vi "FormatInput.vi"(6 "Count to skip":u32, 7 "reset":bool, 8 "valid in":bool, 10 "factor":u16, 11 "data in":T1[](array[typedef])=[{"I"=0.0, "Q"=0.0, "overflow"=FALSE}, {"I"=0.0, "Q"=0.0, "overflow"=FALSE}]) -> (0 "valid out":bool, 3 "Array out":T2)   [LabVIEW 2025]
uses:
  FPGA/subVIs/I32 array size 4.ctl
  <instrlib>/_niInstr/DSP/v1/Shared/Public/IQ Data.ctl
  <instrlib>/_niInstr/DSP/v1/Shared/niInstr DSP v1 Shared.lvlib
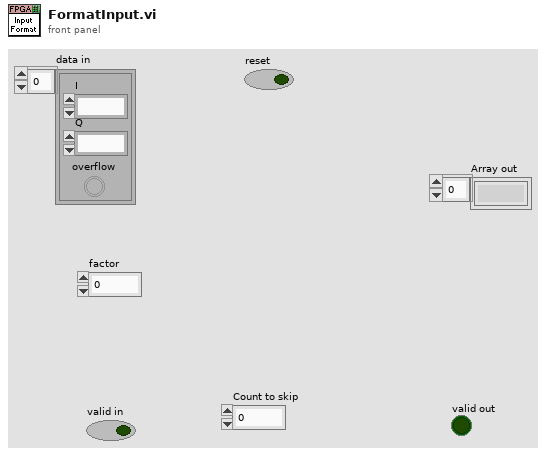
[diagram p1: front panel]
types:
  T1 = typedef "niInstr DSP v1 Shared.lvlib/IQ Data.ctl" = cluster{"I":fxp<+/-,18,1>, "Q":fxp<+/-,18,1>, "overflow":bool}
  T2 = typedef "I32 array size 4.ctl" = fxp<+/-,32,14>[]
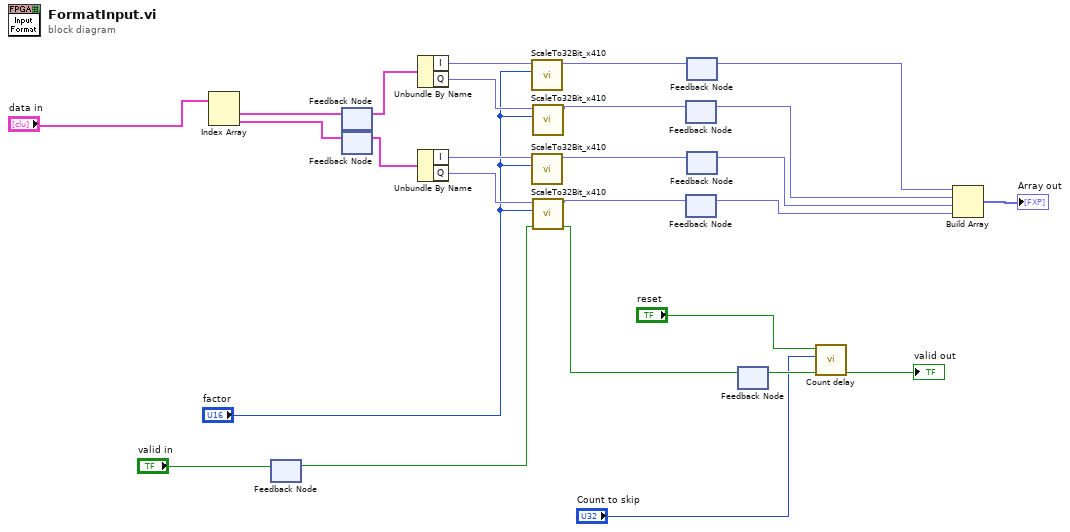
[diagram p0: block diagram]
diagram:
  n1 = Index Array(array="data in") -> (element #1=w26:T1, element #2=w25:T1)  [unwired: 2 in]
  n2 = feedback #1() -> (w8:bool)  [unwired: 1 in]
  n3 = feedback-in #1("valid in") -> ()
  n4 = feedback #2() -> (w19:T1)  [unwired: 1 in]
  n5 = feedback-in #2(w26) -> ()
  n6 = feedback #3() -> (w9:T1)  [unwired: 1 in]
  n7 = feedback-in #3(w25) -> ()
  n8 = Unbundle By Name(w19) -> ("I"=w18:fxp<+/-,18,1>, "Q"=w17:fxp<+/-,18,1>)
  n9 = Unbundle By Name(w9) -> ("I"=w11:fxp<+/-,18,1>, "Q"=w12:fxp<+/-,18,1>)
  n10 = call "ScaleTo32Bit_x410.vi"("factor"="factor", "val"=w18) -> ("32 bit fxp"=w16:fxp<+/-,32,14>)  [unwired: 8 in, 1 out]
  n11 = call "ScaleTo32Bit_x410.vi"("factor"="factor", "val"=w11) -> ("32 bit fxp"=w13:fxp<+/-,32,14>)  [unwired: 8 in, 1 out]
  n12 = call "ScaleTo32Bit_x410.vi"("factor"="factor", "val"=w17) -> ("32 bit fxp"=w15:fxp<+/-,32,14>)  [unwired: 8 in, 1 out]
  n13 = call "ScaleTo32Bit_x410.vi"("valid in"=w8, "factor"="factor", "val"=w12) -> ("valid out"=w7:bool, "32 bit fxp"=w14:fxp<+/-,32,14>)  [unwired: 7 in]
  n14 = feedback #4() -> (w24:fxp<+/-,32,14>)  [unwired: 1 in]
  n15 = feedback-in #4(w15) -> ()
  n16 = feedback #5() -> (w5:fxp<+/-,32,14>)  [unwired: 1 in]
  n17 = feedback-in #5(w14) -> ()
  n18 = feedback #6() -> (w23:fxp<+/-,32,14>)  [unwired: 1 in]
  n19 = feedback-in #6(w16) -> ()
  n20 = feedback #7() -> (w6:fxp<+/-,32,14>)  [unwired: 1 in]
  n21 = feedback-in #7(w13) -> ()
  n22 = feedback #8() -> (w3:bool)  [unwired: 1 in]
  n23 = feedback-in #8(w7) -> ()
  n24 = call "Count delay.vi"("input valid"=w3, "Count to skip"="Count to skip", "Reset"="reset") -> ("output valid"=→"valid out":bool)  [unwired: 7 in, 1 out]
  n25 = Build Array(w23, w24, w6, w5) -> (→"Array out":fxp<+/-,32,14>[])
